vi "Write PCC Data to Optimization.vi"(7 "PCC Data":T1, 8 "error in":errorcluster, 11 "Generic Optimization in":refnum<class "Generic Optimization.lvclass">) -> (0 "error out":errorcluster, 3 "Generic Optimization out":refnum<class "Generic Optimization.lvclass">)   [LabVIEW 2018, in "Generic Optimization Actor.lvlib" / "Generic Optimization.lvclass"]
uses:
  Generic Optimization.lvclass
  Optimization Controls/PCC Data.ctl
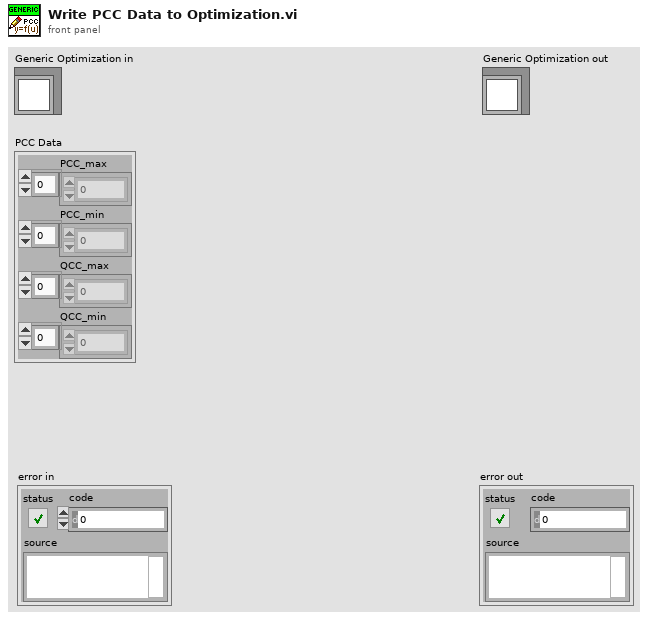
[diagram p1: front panel]
types:
  T1 = typedef "Generic Optimization Actor.lvlib/Generic Optimization.lvclass/PCC Data.ctl" = cluster{"PCC_max":dbl[], "PCC_min":dbl[], "QCC_max":dbl[], "QCC_min":dbl[]}
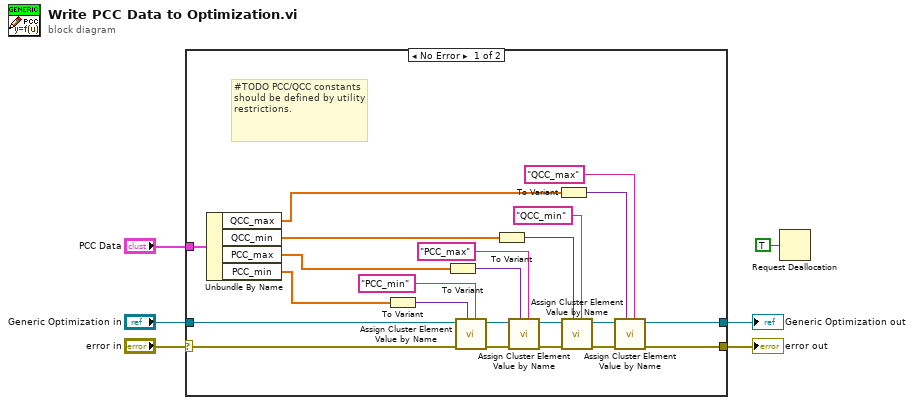
[diagram p0: block diagram]
diagram:
  n1 = case shown="No Error" "error in" {
    selector: "error in" -> [w25 w31]
    tunnel: [w14 w31] -> w6
    tunnel: "Generic Optimization in" -> [w7 w30]
    tunnel: [w8 w30] -> w3
    tunnel: "PCC Data" -> [w13 _]
    frame No Error {
      # "#TODO PCC/QCC constants should be defined by utility restrictions."
      n2 = Unbundle By Name(w13) -> ("QCC_max"=w9:dbl[], "QCC_min"=w10:dbl[], "PCC_max"=w11:dbl[], "PCC_min"=w12:dbl[])
      n3 = To Variant(anything=w12) -> (Variant=w15:variant)
      n4 = To Variant(anything=w11) -> (Variant=w17:variant)
      n5 = call "Assign Cluster Element Value by Name.vi"("Element Name"="PCC_min" ("Keyword Name"), "Value"=w15, "error in"=w25, "Generic Optimization"=w7) -> ("error out"=w19:errorcluster, "Generic Optimization out"=w20:refnum<class "Generic Optimization.lvclass">)  [unwired: 6 in]
      n6 = To Variant(anything=w10) -> (Variant=w21:variant)
      n7 = call "Assign Cluster Element Value by Name.vi"("Element Name"="PCC_max" ("Keyword Name"), "Value"=w17, "error in"=w19, "Generic Optimization"=w20) -> ("error out"=w27:errorcluster, "Generic Optimization out"=w26:refnum<class "Generic Optimization.lvclass">)  [unwired: 6 in]
      n8 = To Variant(anything=w9) -> (Variant=w23:variant)
      n9 = call "Assign Cluster Element Value by Name.vi"("Element Name"="QCC_min" ("Keyword Name"), "Value"=w21, "error in"=w27, "Generic Optimization"=w26) -> ("error out"=w29:errorcluster, "Generic Optimization out"=w28:refnum<class "Generic Optimization.lvclass">)  [unwired: 6 in]
      n10 = call "Assign Cluster Element Value by Name.vi"("Element Name"="QCC_max" ("Keyword Name"), "Value"=w23, "error in"=w29, "Generic Optimization"=w28) -> ("error out"=w14:errorcluster, "Generic Optimization out"=w8:refnum<class "Generic Optimization.lvclass">)  [unwired: 6 in]
    }
    frame Error {
    }
  }
  "error out" <- w6
  "Generic Optimization out" <- w3
  n11 = Request Deallocation(TRUE ("flag")) -> ()
